vi "Configuration 1.4 JSON Flatten.vi"(8 "error in (no error)":errorcluster, 11 "configuration 1.4":T2={"plugins"=[{"core"={"name"="", "components"=[], "cycle timing"={"priority"=10000, "decimation"=1, "offset"=0}}, "component settings"=[], "threads"=[{"core"={"processor"=-2, "priority offset"=0}, "component settings"=[], "transfer groups"=[{"core"={"name"="Group", "direction"=0, "cycle timing"={"priority"=100, "decimation"=1, "offset"=0}, "timeout behavior"=0, "enable conversion"=FALSE}, "component settings"=[], "transfers"=[{"core"={"name"="Transfer"}, "component settings"=[], "channels"=[{"core"={"name"="Channel", "units"="V", "engine data type"=2, "string data type"=2, "string offset"=0}, "component settings"=[]}]}]}]}]}]}) -> (0 "error out":errorcluster, 2 "dsf version":T1, 3 "dsf configuration json":string)   [LabVIEW 2019, in "DSF Core.lvlib" / "Configuration Session.lvclass"]
uses:
  Configuration Session.lvclass
  Typedefs/DSF Version Info.ctl
  DSF Core.lvlib
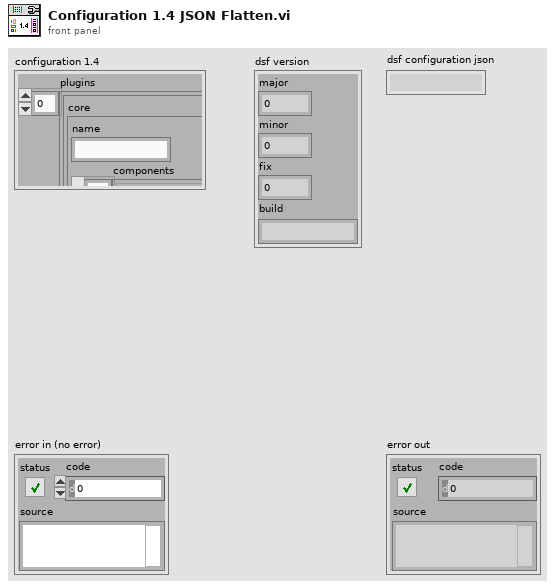
[diagram p1: front panel]
types:
  T1 = typedef "DSF Core.lvlib/DSF Version Info.ctl" = cluster{"major":u32, "minor":u32, "fix":u32, "build":string}
  T2 = cluster{"plugins":cluster{"core":cluster{"name":string, "components":string[], "cycle timing":cluster{"priority":u64, "decimation":u64, "offset":u64}}, "component settings":cluster{"component":string, "values":cluster{"key":string, "value":string}[]}[], "threads":cluster{"core":cluster{"processor":i32, "priority offset":i16}, "component settings":cluster{"component":string, "values":cluster{"key":string, "value":string}[]}[], "transfer groups":cluster{"core":cluster{"name":string, "direction":i32, "cycle timing":cluster{"priority":u64, "decimation":u64, "offset":u64}, "timeout behavior":u8, "enable conversion":bool}, "component settings":cluster{"component":string, "values":cluster{"key":string, "value":string}[]}[], "transfers":cluster{"core":cluster{"name":string}, "component settings":cluster{"component":string, "values":cluster{"key":string, "value":string}[]}[], "channels":cluster{"core":cluster{"name":string, "units":string, "engine data type":u8, "string data type":u8, "string offset":u64}, "component settings":cluster{"component":string, "values":cluster{"key":string, "value":string}[]}[]}[]}[]}[]}[]}[]}
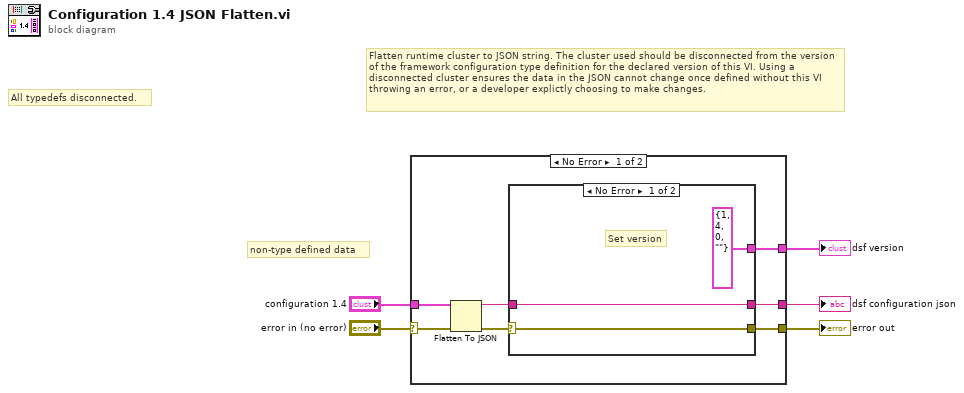
[diagram p0: block diagram]
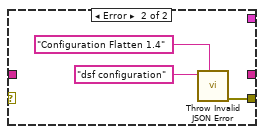
[diagram p2: hidden frame]
diagram:
  # "non-type defined data"
  # "All typedefs disconnected."
  # "Flatten runtime cluster to JSON string. The cluster used should be disconnected from the version of the framework configuration type definition for the declared version of this VI. Using a disconnected cluster ensures the data in the JSON cannot change once defined without this VI throwing an error, or a developer explictly choosing to make changes."
  n1 = case shown="No Error" "error in (no error)" {
    selector: "error in (no error)" -> [w9 w19]
    tunnel: [w11 w19] -> w5
    tunnel: "configuration 1.4" -> [w6 _]
    tunnel: [w8 _] -> w2
    tunnel: [w7 _] -> w1
    frame No Error {
      n2 = Flatten To JSON(anything=w6, error in (no error)=w9) -> (JSON string=w10:string, 11:w12:errorcluster)  [unwired: 1 in]
      n3 = case shown="No Error" w12 {
        selector: w12 -> [w15 _]
        tunnel: [w15 w18] -> w11
        tunnel: w10 -> [w14 _]
        tunnel: [w14 _] -> w8
        tunnel: [T1 {"major"=1, "minor"=4, "fix"=0, "build"=""} ("json version") _] -> w7
        frame No Error {
          # "Set version"
        }
        frame Error {
          n4 = call "Throw Invalid JSON Error.vi"("error source vi name"="Configuration Flatten 1.4", "name"="dsf configuration") -> ("error out"=w18:errorcluster)  [unwired: 9 in]
        }
      }
    }
    frame Error {
    }
  }
  "dsf configuration json" <- w2
  "error out" <- w5
  "dsf version" <- w1
